vi "Controller - Fire Stop.vi"(8 "error in (no error)":errorcluster, 10 "Stop?":bool, 11 "View Model":T1) -> (0 "error out":errorcluster)   [LabVIEW 2017]
doc: "Generate Stop command and store into DVR to terminate all process"
uses:
  View Model/Controls/View Model.ctl
  View Model/Controls/Shared Model.ctl
  Error Handler/Controls/Error Model.ctl
  Error Handler/Controls/Error Event.ctl
  Error Handler/Controls/Error Type.ctl
  Controls/Controller Model.ctl
  Controls/Controller Event.ctl
  Controls/Controller Command.ctl
  Controls/Controller Overhead.ctl
  Real-Time/RT Status.ctl
  Real-Time/RT Loop Status.ctl
  Controls/Controller NStream.ctl
  Controls/Controller DAQ Data.ctl
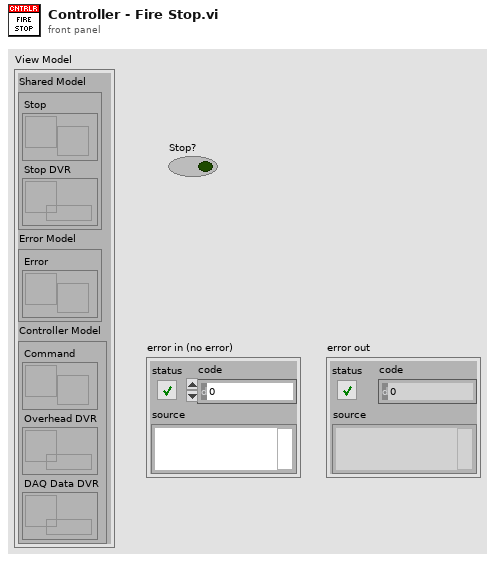
[diagram p1: front panel]
types:
  T1 = typedef "View Model.ctl" = cluster{"Shared Model":T2, "Error Model":T3, "Controller Model":T4}
  T2 = typedef "Shared Model.ctl" = cluster{"Stop":refnum<user-event>, "Stop DVR":refnum<data-value>}
  T3 = typedef "Error Model.ctl" = cluster{"Error":refnum<user-event>}
  T4 = typedef "Controller Model.ctl" = cluster{"Command":refnum<user-event>, "Overhead DVR":refnum<data-value>, "DAQ Data DVR":refnum<data-value>}
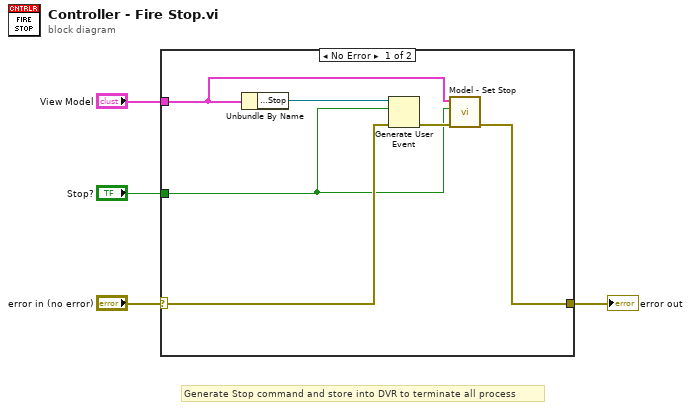
[diagram p0: block diagram]
diagram:
  # "Generate Stop command and store into DVR to terminate all process"
  n1 = case shown="No Error" "error in (no error)" {
    selector: "error in (no error)" -> [w9 w11]
    tunnel: [w5 w11] -> w3
    tunnel: "View Model" -> [w6 _]
    tunnel: "Stop?" -> [w7 _]
    frame No Error {
      n2 = Unbundle By Name(w6) -> ("Shared Model.Stop"=w10:refnum<user-event>)
      n3 = Generate User Event(user event=w10, event data cluster=w7, error in=w9) -> (error out=w8:errorcluster)  [unwired: 1 in, 1 out]
      n4 = call "Model - Set Stop.vi"("error in (no error)"=w8, "Stop"=w7, "View Model"=w6) -> ("error out"=w5:errorcluster)  [unwired: 7 in, 1 out]
    }
    frame Error {
    }
  }
  "error out" <- w3
